vi "Teleop.vi"(10 "Match Info":T1={"Autonomous Elapsed Seconds"=0.0, "TeleOp Elapsed Seconds"=0.0, "Disabled Elapsed Seconds"=0.0, "Visited Autonomous"=FALSE, "Visited TeleOp"=FALSE, "Visited Disabled"=FALSE, "Autonomous Settings"={"Autonomous Style"=enum."Independent", "VI Refnum"=refnum}}, 11 "Call Context":T2) -> ()   [LabVIEW 2017]
doc: "This VI is called for each TeleOp packet received from the DS where the robot is not disabled. It is often used to read from the joysticks and update I/O or to update setpoints for timed control loops. It should complete and return within 20 milliseconds or it may miss DS packets."
uses:
  <vilib>/Rock Robotics/WPI/DriverStation/WPI_DriverStationDerivedRobotMode.ctl
  <vilib>/Rock Robotics/WPI/DriverStation/WPI_DriverStationMatch Info.ctl
  <vilib>/Rock Robotics/WPI/Solenoid/WPI_SolenoidValue.ctl
  <vilib>/Rock Robotics/WPI/Utilities/WPI_GetSetVariantRefNum.vi
  <vilib>/Rock Robotics/Network Tables/NT Write Numeric Array.vi
  <vilib>/Rock Robotics/Network Tables/NT Read Boolean.vi
  <vilib>/Rock Robotics/Network Tables/NT Read Number.vi
  <vilib>/Rock Robotics/Network Tables/NT Write Boolean Array.vi
  <vilib>/Rock Robotics/WPI/Solenoid/WPI_SolenoidSetEnum.vi
  <vilib>/addons/control/pid/pid.llb/PID (DBL).vi
  <vilib>/addons/control/pid/NI_PID_pid.lvlib
panel:
  out "Sample Slider 1":dbl(slide) scale=0.0..5.0
  out "Sample Boolean 3":bool
  out "Sample Boolean 2":bool
  out "Sample Slider 0":dbl(slide) scale=0.0..5.0
  out "Sample Boolean 1":bool
  out "Sample Boolean 0":bool
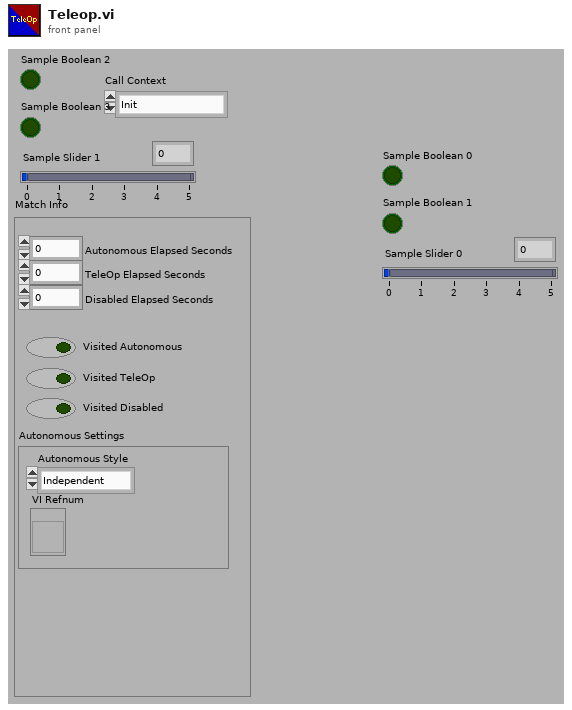
[diagram p1: front panel]
types:
  T1 = typedef "WPI_DriverStationMatch Info.ctl" = cluster{"Autonomous Elapsed Seconds":dbl, "TeleOp Elapsed Seconds":dbl, "Disabled Elapsed Seconds":dbl, "Visited Autonomous":bool, "Visited TeleOp":bool, "Visited Disabled":bool, "Autonomous Settings":cluster{"Autonomous Style":enum16{"Iterative", "Independent"}, "VI Refnum":refnum<vi>}}
  T2 = typedef "WPI_DriverStationDerivedRobotMode.ctl" = enum16{"Init", "Execute", "Stop"}
  T3 = cluster{"proportional gain (Kc)":dbl, "integral time (Ti, min)":dbl, "derivative time (Td, min)":dbl}
  T4 = typedef "WPI_SolenoidValue.ctl" = enum16{"Off", "On", "Forward", "Reverse"}
  T5 = typedef "WPI_JoystickDevRef.ctl" = cluster{"Device":T6}
  T6 = typedef "WPI_JoystickDeviceEnum.ctl" = enum16{"USB 0", "USB 1", "USB 2", "USB 3", "USB 4", "USB 5"}
  T7 = typedef "WPI_DigitalInputDevRef.ctl" = cluster{"DevStatus":errorcluster, "DIO Channel":T8}
  T8 = typedef "FPGA_DIOChannel.ctl" = enum8{"DIO 0", "DIO 1", "DIO 2", "DIO 3", "DIO 4", "DIO 5", "DIO 6", "DIO 7", "DIO 8", "DIO 9", "DIO MXP 0", "DIO MXP 1", "DIO MXP 2", "DIO MXP 3", "DIO MXP 4", "DIO MXP 5", "DIO MXP 6", "DIO MXP 7", "DIO MXP 8", "DIO MXP 9", "DIO MXP 10", "DIO MXP 11", "DIO MXP 12", "DIO MXP 13", "DIO MXP 14", "DIO MXP 15", "SPI Port CS1", "SPI Port CS2", "SPI Port CS3", "SPI Port MISO", "SPI Port MOSI", "Invalid"}
  T9 = typedef "WPI_RobotDriveDevRef.ctl" = cluster{"DevStatus":errorcluster, "Motors[]":T10[], "Square Inputs":bool, "Max Output":dbl}
  T10 = typedef "WPI_MotorControlDeviceRef.ctl" = cluster{"DeviceStatus":errorcluster, "Type":T11, "PWM":cluster{"PWM Channel":T12, "DeadBand":T13}, "CAN":cluster{"Device Number":u8, "SetOutput VI Ref":variant, "GetOutput VI Ref":variant, "Enable VI Ref":variant, "Disable VI Ref":variant, "Data":variant}, "Invert":bool, "DIO PWM":cluster{"PWM \"Enable\" Channel":T12, "DIOChannel":T8, "PWM Rate":dbl}}
  T11 = typedef "WPI_MotorControlType.ctl" = enum16{"PWM", "CAN", "DIO PWM"}
  T12 = typedef "FPGA_DIOPWMChannel.ctl" = enum8{"PWM 0", "PWM 1", "PWM 2", "PWM 3", "PWM 4", "PWM 5", "PWM 6", "PWM 7", "PWM 8", "PWM 9", "PWM MXP 0", "PWM MXP 1", "PWM MXP 2", "PWM MXP 3", "PWM MXP 4", "PWM MXP 5", "PWM MXP 6", "PWM MXP 7", "PWM MXP 8", "PWM MXP 9", "Invalid"}
  T13 = typedef "WPI_PWMDeadband.ctl" = cluster{"Name":string, "maxPositivePwm":i32, "minPositivePwm":i32, "centerPwm":i32, "maxNegativePwm":i32, "minNegativePwm":i32, "angularRange":u16}
  T14 = typedef "WPI_EncoderDevRef.ctl" = cluster{"DevStatus":errorcluster, "EncoderIndex":T15, "CounterIndex":T16, "DistancePerCount":dbl, "Decoding Type":T17}
  T15 = typedef "FPGA_EncoderIdx.ctl" = enum8{"Enc 0", "Enc 1", "Enc 2", "Enc 3", "Enc 4", "Enc 5", "Enc 6", "Enc 7", "Invalid"}
  T16 = typedef "FPGA_CounterCtrSystemIndex.ctl" = enum8{"Ctr 0", "Ctr 1", "Ctr 2", "Ctr 3", "Ctr 4", "Ctr 5", "Ctr 6", "Ctr 7", "Invalid"}
  T17 = typedef "WPI_EncoderType.ctl" = enum16{"1x", "2x", "4x"}
  T18 = typedef "WPI_SolenoidDevRef.ctl" = cluster{"DevStatus":errorcluster, "Pneumatics Control Module":u8, "Forward Solenoid Channel":T19, "Reverse Solenoid Channel":T19}
  T19 = typedef "WPI_SolenoidChannel.ctl" = enum8{"Solenoid 0", "Solenoid 1", "Solenoid 2", "Solenoid 3", "Solenoid 4", "Solenoid 5", "Solenoid 6", "Solenoid 7", "Invalid"}
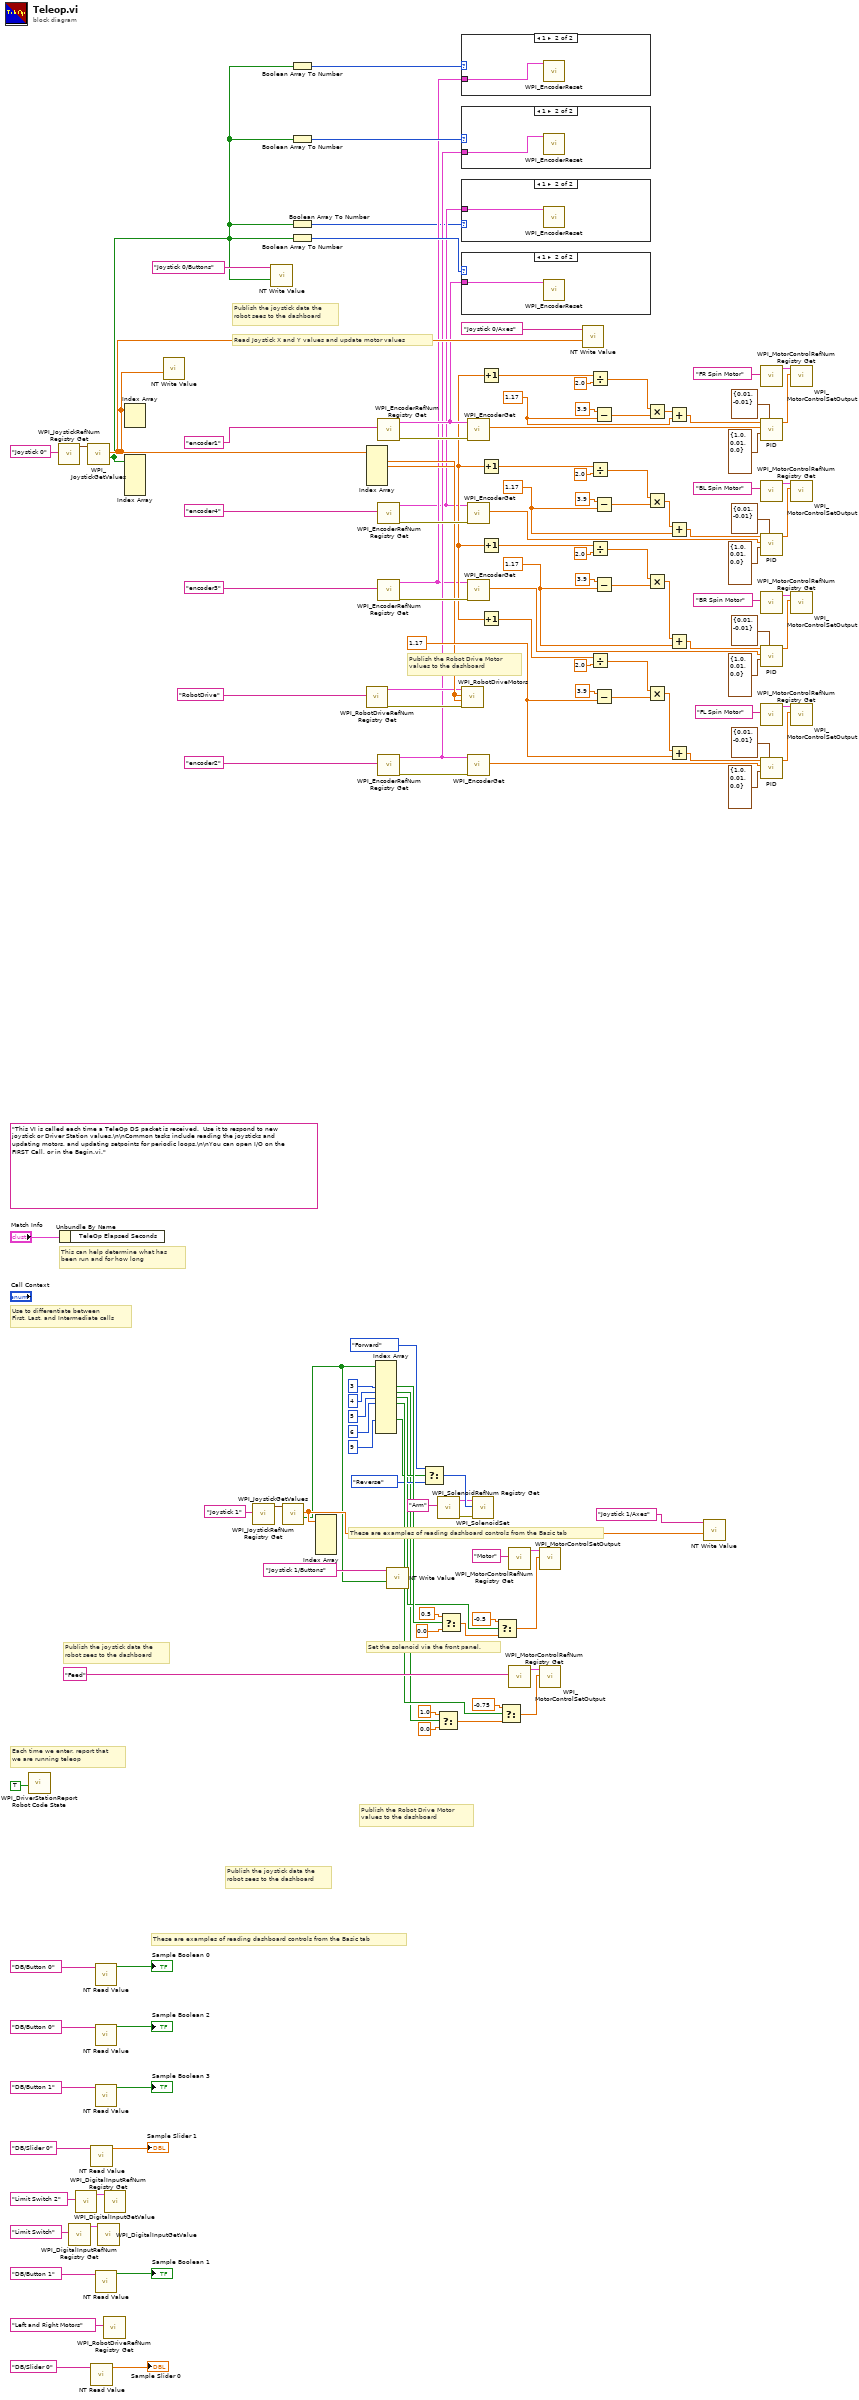
[diagram p0: block diagram]
diagram:
  w25 = 1.17 ("y")
  w41 = 1.17 ("y")
  w57 = 1.17 ("y")
  w73 = 1.17 ("y")
  (unwired) "This VI is called each time a TeleOp DS packet is received.  Use it to respond to new joystick or Driver Station values.\n\nCommon tasks include reading the joysticks and updating motors, and updating setpoints for periodic loops.\n\nYou can open I/O on the FIRST Call, or in the Begin.vi."
  # "Set the solenoid via the front panel."
  # "Publish the joystick data the\nrobot sees to the dashboard"
  # "These are examples of reading dashboard controls from the Basic tab"
  # "Publish the Robot Drive Motor\nvalues to the dashboard"
  # "Publish the joystick data the\nrobot sees to the dashboard"
  # "These are examples of reading dashboard controls from the Basic tab"
  # "Publish the Robot Drive Motor\nvalues to the dashboard"
  # "Publish the joystick data the\nrobot sees to the dashboard"
  # "Each time we enter, report that\nwe are running teleop"
  # "Use to differentiate between\nFirst, Last, and Intermediate calls"
  # "This can help determine what has\nbeen run and for how long"
  # "Read Joystick X and Y values and update motor values"
  n1 = call <vilib>:"WPI_DriverStationReport Robot Code State.vi"("TeleOp"=TRUE ("Autonomous")) -> ()  [unwired: 10 in, 1 out]
  n2 = call <vilib>:"WPI_JoystickRefNum Registry Get.vi"("refnum name"="Joystick 0") -> ("JoystickDevRef"=w135:T5)  [unwired: 1 in, 9 out]
  n3 = Unbundle By Name("Match Info") -> ()  [unwired: 1 out]
  n4 = call <vilib>:"WPI_DigitalInputRefNum Registry Get.vi"("refnum name"="Limit Switch") -> ("DigitalInputDevRef"=w104:T7)  [unwired: 9 in, 1 out]
  n5 = call <vilib>:"WPI_DigitalInputRefNum Registry Get.vi"("refnum name"="Limit Switch 2") -> ("DigitalInputDevRef"=w102:T7)  [unwired: 9 in, 1 out]
  n6 = call <vilib>:"WPI_JoystickGetValues.vi"("JoystickDevRef"=w135) -> ("Buttons"=w1:bool[], "Axes"=w14:dbl[])  [unwired: 6 in, 3 out]
  n7 = call-poly <vilib>:"NT Read Value.vi"("Name"="DB/Slider 0" ("refnum name")) -> ("Numeric"=→"Sample Slider 1":dbl)  [unwired: 9 in, 1 out]
  n8 = call-poly <vilib>:"NT Read Value.vi"("Name"="DB/Slider 0" ("refnum name")) -> ("Numeric"=→"Sample Slider 0":dbl)  [unwired: 9 in, 1 out]
  n9 = call-poly <vilib>:"NT Read Value.vi"("Name"="DB/Button 0" ("refnum name")) -> ("Boolean"=→"Sample Boolean 0":bool)  [unwired: 9 in, 1 out]
  n10 = call-poly <vilib>:"NT Read Value.vi"("Name"="DB/Button 0" ("refnum name")) -> ("Boolean"=→"Sample Boolean 2":bool)  [unwired: 9 in, 1 out]
  n11 = call-poly <vilib>:"NT Read Value.vi"("Name"="DB/Button 1" ("refnum name")) -> ("Boolean"=→"Sample Boolean 3":bool)  [unwired: 9 in, 1 out]
  n12 = call-poly <vilib>:"NT Read Value.vi"("Name"="DB/Button 1" ("refnum name")) -> ("Boolean"=→"Sample Boolean 1":bool)  [unwired: 9 in, 1 out]
  n13 = call <vilib>:"WPI_DigitalInputGetValue.vi"("DigitalInputDevRef"=w104) -> ()  [unwired: 8 in, 3 out]
  n14 = call <vilib>:"WPI_RobotDriveRefNum Registry Get.vi"("refnum name"="Left and Right Motors") -> ()  [unwired: 1 in, 10 out]
  n15 = call <vilib>:"WPI_DigitalInputGetValue.vi"("DigitalInputDevRef"=w102) -> ()  [unwired: 8 in, 3 out]
  n16 = Index Array(array=w14) -> ()  [unwired: 2 in, 2 out]
  n17 = Index Array(array=w1) -> ()  [unwired: 5 in, 5 out]
  n18 = call-poly <vilib>:"NT Write Value.vi"("Numeric Array"=w14) -> ()  [unwired: 10 in, 1 out]
  n19 = call <vilib>:"WPI_JoystickRefNum Registry Get.vi"("refnum name"="Joystick 1") -> ("JoystickDevRef"=w96:T5)  [unwired: 1 in, 9 out]
  n20 = call-poly <vilib>:"NT Write Value.vi"("Boolean Array"=w1, "Name"="Joystick 0/Buttons") -> ()  [unwired: 9 in, 1 out]
  n21 = call <vilib>:"WPI_JoystickGetValues.vi"("JoystickDevRef"=w96) -> ("Buttons"=w94:bool[], "Axes"=w95:dbl[])  [unwired: 6 in, 3 out]
  n22 = Boolean Array To Number(Boolean array=w1) -> (number=w4:u32)
  n23 = Boolean Array To Number(Boolean array=w1) -> (number=w7:u32)
  n24 = Boolean Array To Number(Boolean array=w1) -> (number=w2:u32)
  n25 = Boolean Array To Number(Boolean array=w1) -> (number=w9:u32)
  n26 = Index Array(array=w95) -> ()  [unwired: 5 in, 5 out]
  n27 = Index Array(array=w14) -> (element #1=w13:dbl, element #2=w8:dbl)  [unwired: 5 in, 3 out]
  n28 = call <vilib>:"WPI_RobotDriveRefNum Registry Get.vi"("refnum name"="RobotDrive") -> ("error out"=w11:errorcluster, "RobotDriveDevRef"=w12:T9)  [unwired: 1 in, 8 out]
  n29 = Index Array(array=w94, index #3=3 ("index"), index #4=4 ("index"), index #5=5 ("index"), index #6=6 ("index"), index #9=9 ("index")) -> (element #3=w100:bool, element #4=w80:bool, element #5=w84:bool, element #6=w107:bool, element #9=w85:bool)  [unwired: 6 in, 6 out]
  n30 = call <vilib>:"WPI_EncoderRefNum Registry Get.vi"("refnum name"="encoder1") -> ("error out"=w68:errorcluster, "EncoderDevRef"=w10:T14)  [unwired: 9 in]
  n31 = call <vilib>:"WPI_EncoderRefNum Registry Get.vi"("refnum name"="encoder4") -> ("error out"=w20:errorcluster, "EncoderDevRef"=w3:T14)  [unwired: 9 in]
  n32 = call <vilib>:"WPI_EncoderRefNum Registry Get.vi"("refnum name"="encoder3") -> ("error out"=w36:errorcluster, "EncoderDevRef"=w5:T14)  [unwired: 9 in]
  n33 = call <vilib>:"WPI_EncoderRefNum Registry Get.vi"("refnum name"="encoder2") -> ("error out"=w52:errorcluster, "EncoderDevRef"=w6:T14)  [unwired: 9 in]
  n34 = call-poly <vilib>:"NT Write Value.vi"("Boolean Array"=w94, "Name"="Joystick 1/Buttons") -> ()  [unwired: 9 in, 1 out]
  n35 = Select(t=WPI_SolenoidValue."Forward" ("Value"), s=w85, f=WPI_SolenoidValue."Reverse") -> (s? t:f=w89:T4)
  n36 = Select(t=1.0, s=w80, f=0.0) -> (s? t:f=w110:dbl)
  n37 = call <vilib>:"WPI_SolenoidRefNum Registry Get.vi"("refnum name"="Arm") -> ("error out"=w87:errorcluster, "SolenoidDevRef"=w88:T18)  [unwired: 9 in]
  n38 = Select(t=0.5, s=w100, f=0.0) -> (s? t:f=w99:dbl)
  n39 = case shown="1" w4 {
    tunnel: w5 -> [_ w139]
    frame 0, Default {
    }
    frame 1 {
      n40 = call <vilib>:"WPI_EncoderReset.vi"("EncoderDevRef"=w139) -> ()  [unwired: 9 in, 2 out]
    }
  }
  n41 = case shown="1" w7 {
    tunnel: w6 -> [_ w140]
    frame 0, Default {
    }
    frame 1 {
      n42 = call <vilib>:"WPI_EncoderReset.vi"("EncoderDevRef"=w140) -> ()  [unwired: 9 in, 2 out]
    }
  }
  n43 = case shown="1" w2 {
    tunnel: w3 -> [_ w141]
    frame 0, Default {
    }
    frame 1 {
      n44 = call <vilib>:"WPI_EncoderReset.vi"("EncoderDevRef"=w141) -> ()  [unwired: 9 in, 2 out]
    }
  }
  n45 = case shown="1" w9 {
    tunnel: w10 -> [_ w142]
    frame 0, Default {
    }
    frame 1 {
      n46 = call <vilib>:"WPI_EncoderReset.vi"("EncoderDevRef"=w142) -> ()  [unwired: 9 in, 2 out]
    }
  }
  n47 = call <vilib>:"WPI_RobotDriveMotors.vi"("error in (no error)"=w11, "RightSpeed"=w13, "LeftSpeed"=w13, "RobotDriveDevRef"=w12) -> ()  [unwired: 5 in, 3 out]
  n48 = call <vilib>:"WPI_EncoderGet.vi"("error in (no error)"=w68, "EncoderDevRef"=w10) -> ("Distance"=w69:dbl)  [unwired: 4 in, 5 out]
  n49 = call <vilib>:"WPI_EncoderGet.vi"("error in (no error)"=w20, "EncoderDevRef"=w3) -> ("Distance"=w21:dbl)  [unwired: 4 in, 5 out]
  n50 = call <vilib>:"WPI_EncoderGet.vi"("error in (no error)"=w36, "EncoderDevRef"=w5) -> ("Distance"=w37:dbl)  [unwired: 4 in, 5 out]
  n51 = call <vilib>:"WPI_EncoderGet.vi"("error in (no error)"=w52, "EncoderDevRef"=w6) -> ("Distance"=w53:dbl)  [unwired: 4 in, 5 out]
  n52 = call-poly <vilib>:"WPI_SolenoidSet.vi"("error in (no error)"=w87, "Value"=w89, "SolenoidDevRef"=w88) -> ()  [unwired: 9 out]
  n53 = Increment(x=w8) -> (x+1=w78:dbl)
  n54 = Increment(x=w8) -> (x+1=w30:dbl)
  n55 = Increment(x=w8) -> (x+1=w46:dbl)
  n56 = Increment(x=w8) -> (x+1=w62:dbl)
  n57 = Select(t=-0.5, s=w84, f=w99) -> (s? t:f=w93:dbl)
  n58 = Select(t=-0.75, s=w107, f=w110) -> (s? t:f=w113:dbl)
  n59 = call <vilib>:"WPI_MotorControlRefNum Registry Get.vi"("refnum name"="Motor") -> ("MotorControlDevRef"=w106:T10)  [unwired: 9 in, 1 out]
  n60 = call <vilib>:"WPI_MotorControlRefNum Registry Get.vi"("refnum name"="Feed") -> ("MotorControlDevRef"=w112:T10)  [unwired: 9 in, 1 out]
  n61 = call <vilib>:"WPI_MotorControlSetOutput.vi"("Output"=w93, "MotorControlDevRef"=w106) -> ()  [unwired: 7 in, 3 out]
  n62 = call <vilib>:"WPI_MotorControlSetOutput.vi"("Output"=w113, "MotorControlDevRef"=w112) -> ()  [unwired: 7 in, 3 out]
  n63 = call-poly <vilib>:"NT Write Value.vi"("Numeric Array"=w14, "Name"="Joystick 0/Axes") -> ()  [unwired: 9 in, 1 out]
  n64 = Divide(x=w78, y=2.0) -> (x/y=w76:dbl)
  n65 = Divide(x=w30, y=2.0) -> (x/y=w28:dbl)
  n66 = Divide(x=w46, y=2.0) -> (x/y=w44:dbl)
  n67 = Divide(x=w62, y=2.0) -> (x/y=w60:dbl)
  n68 = Subtract(x=3.9, y=w73) -> (x-y=w75:dbl)
  n69 = Subtract(x=3.9, y=w25) -> (x-y=w27:dbl)
  n70 = Subtract(x=3.9, y=w41) -> (x-y=w43:dbl)
  n71 = Subtract(x=3.9, y=w57) -> (x-y=w59:dbl)
  n72 = Multiply(x=w76, y=w75) -> (x*y=w72:dbl)
  n73 = Multiply(x=w28, y=w27) -> (x*y=w24:dbl)
  n74 = Multiply(x=w44, y=w43) -> (x*y=w40:dbl)
  n75 = Multiply(x=w60, y=w59) -> (x*y=w56:dbl)
  n76 = Add(x=w72, y=w73) -> (x+y=w71:dbl)
  n77 = Add(x=w24, y=w25) -> (x+y=w23:dbl)
  n78 = Add(x=w40, y=w41) -> (x+y=w39:dbl)
  n79 = Add(x=w56, y=w57) -> (x+y=w55:dbl)
  n80 = call-poly <vilib>:"NT Write Value.vi"("Numeric Array"=w95, "Name"="Joystick 1/Axes") -> ()  [unwired: 9 in, 1 out]
  n81 = call <vilib>:"WPI_MotorControlRefNum Registry Get.vi"("refnum name"="FR Spin Motor") -> ("MotorControlDevRef"=w65:T10)  [unwired: 9 in, 1 out]
  n82 = call-poly <vilib>:"PID.vi"("output range"=cluster{"output high":dbl, "output low":dbl} {"output high"=0.01, "output low"=-0.01}, "PID gains"=T3 {"proportional gain (Kc)"=1.0, "integral time (Ti, min)"=0.01, "derivative time (Td, min)"=0.0}, "process variable"=w69, "setpoint"=w71) -> ("output"=w66:dbl)  [unwired: 6 in, 1 out]
  n83 = call <vilib>:"WPI_MotorControlRefNum Registry Get.vi"("refnum name"="BL Spin Motor") -> ("MotorControlDevRef"=w17:T10)  [unwired: 9 in, 1 out]
  n84 = call-poly <vilib>:"PID.vi"("output range"=cluster{"output high":dbl, "output low":dbl} {"output high"=0.01, "output low"=-0.01}, "PID gains"=T3 {"proportional gain (Kc)"=1.0, "integral time (Ti, min)"=0.01, "derivative time (Td, min)"=0.0}, "process variable"=w21, "setpoint"=w23) -> ("output"=w18:dbl)  [unwired: 6 in, 1 out]
  n85 = call <vilib>:"WPI_MotorControlRefNum Registry Get.vi"("refnum name"="BR Spin Motor") -> ("MotorControlDevRef"=w33:T10)  [unwired: 9 in, 1 out]
  n86 = call-poly <vilib>:"PID.vi"("output range"=cluster{"output high":dbl, "output low":dbl} {"output high"=0.01, "output low"=-0.01}, "PID gains"=T3 {"proportional gain (Kc)"=1.0, "integral time (Ti, min)"=0.01, "derivative time (Td, min)"=0.0}, "process variable"=w37, "setpoint"=w39) -> ("output"=w34:dbl)  [unwired: 6 in, 1 out]
  n87 = call <vilib>:"WPI_MotorControlRefNum Registry Get.vi"("refnum name"="FL Spin Motor") -> ("MotorControlDevRef"=w49:T10)  [unwired: 9 in, 1 out]
  n88 = call-poly <vilib>:"PID.vi"("output range"=cluster{"output high":dbl, "output low":dbl} {"output high"=0.01, "output low"=-0.01}, "PID gains"=T3 {"proportional gain (Kc)"=1.0, "integral time (Ti, min)"=0.01, "derivative time (Td, min)"=0.0}, "process variable"=w53, "setpoint"=w55) -> ("output"=w50:dbl)  [unwired: 6 in, 1 out]
  n89 = call <vilib>:"WPI_MotorControlSetOutput.vi"("Output"=w66, "MotorControlDevRef"=w65) -> ()  [unwired: 7 in, 3 out]
  n90 = call <vilib>:"WPI_MotorControlSetOutput.vi"("Output"=w18, "MotorControlDevRef"=w17) -> ()  [unwired: 7 in, 3 out]
  n91 = call <vilib>:"WPI_MotorControlSetOutput.vi"("Output"=w34, "MotorControlDevRef"=w33) -> ()  [unwired: 7 in, 3 out]
  n92 = call <vilib>:"WPI_MotorControlSetOutput.vi"("Output"=w50, "MotorControlDevRef"=w49) -> ()  [unwired: 7 in, 3 out]
